vi "DefenderNormalNova.vi"(0 "Enum":T1(ring)=enum."Marcar o mais perigoso", 1 "Atacando contra?":bool=TRUE, 3 "AI Parameters":T9={"GotoKick"={"Dist do cone a frente"=150.0, "attacker farback"=1500.0, "Perto"=300.0, "min dist to kick"=150.0, "kick eps"=0.0, "Time to transition"=0.05}, "Attacker"={"CC chute"=0.09, "CC passe"=0.045, "Kick Force"=100.0, "D ball-robot Kick"=200.0, "D ball-robot Pass"=0.3}, "Defender"={"D max"=1700.0, "Vel p/ robô av"=1000.0, "Kick Force"=100.0, "D atk-def"=0.0, "D farback"=0.0}, "Timeout"={"Field/v in x"=6.0, "Dist Robots"=300, "Dist up in y"=300}, "Pose Striker"={"dist"=200.0, "Numeric"=-4.0, "dist 2"=200.0}, "Dist Stop"=300.0, "Distance when ball out"=200, "D central gap "=150.0, "T pass"=0.0, "Force ++"=0.0, "range kick"=0.0, "Chute alto"=TRUE, "Marcador novo"=TRUE} {"D central gap" format="%#_13g"; "Dist Stop" format="%#_13g"; "Pose Striker"."Numeric" format="%#_13g"; "Defender"."Kick Force" format="%#_13g"; "Defender"."Vel p/ robô av" format="%#_13g"; "Attacker"."D ball-robot Kick" format="%#_13g"; "Attacker"."Kick Force" format="%#_13g"; "Attacker"."CC passe" format="%#_13g"; "Attacker"."CC chute" format="%#_13g"; "GotoKick"."kick eps" format="%#_13g"; "GotoKick"."min dist to kick" format="%#_13g"; "GotoKick"."Perto" format="%#_13g"; "GotoKick"."attacker farback" format="%#_13g"; "GotoKick"."Dist do cone a frente" format="%#_13g"}, 4 "IA State Input 2":T10={"our_robots"=[], "enemy_robots"=[], "balls"=[], "geometry"={"line_width"=0, "field_length"=0, "field_width"=0, "boundary_width"=0, "referee_width"=0, "goal_width"=0, "goal_depth"=0, "goal_wall_width"=0, "center_circle_radius"=0, "defense_radius"=0, "defense_stretch"=0, "free_kick_from_defense_dist"=0, "penalty_spot_from_field_line_dist"=0, "penalty_line_from_spot_dist"=0}, "IA Judge"={"stage"="", "command"="", "our_goalie_id"=0.0, "enemy_goalie_id"=0.0, "command enum"=enum."Halt", "Time"=enum."Azul"}, "Received Timestamp"=timestamp(0 s since 1904-01-01), "Events"={"Touch"=FALSE, "Ball out"=FALSE, "id touch"=0.0, "Ball out of \nVision"=FALSE, "Ball inside \nGoalie area"=FALSE, "Robot not responding"=FALSE, "Robots responding status"=[1.0, 1.0, 1.0, 1.0, 1.0, 1.0], "Enemy Ball \nPossession"=FALSE, "Pass State"=FALSE, "id end of pass"=0.0, "Kick"=FALSE, "Id ini Possession"=0.0, "Ball Possesion"=FALSE, "Id Possesion"=0.0}}, 5 "Stop?":bool, 6 "Defensores":u32[](array[numeric]), 7 "total de \ndefensores":i32, 8 "Field defense":dbl[](array[numeric]), 9 "geometry":T7, 10 "balls":T8[](array[typedef]), 11 "Our Robot":T2={"id"=0, "function"=enum."Attacker", "x"=0.0, "y"=0.0, "orientation"=0.0, "v_tangent"=0.0, "v_normal"=0.0, "v_ang"=0.0, "kick_x"=0.0, "kick_z"=0.0, "dribble"=FALSE, "Timestamp"=timestamp(0 s since 1904-01-01), "estimatives"={"est_v_tangent"=0.0, "est_v_normal"=0.0, "est_vx"=0.0, "est_vy"=0.0, "Pos Robot Est"=[]}, "dest_x_kick"=0.0, "dest_y_kick"=0.0, "Gap Coord"=[], "States"=enum."GoToTangent", "Path "=[], "Path  Smooth"=[], "Dest"=[]}) -> (2 "Robot out":T2={"id"=0, "function"=enum."Attacker", "x"=0.0, "y"=0.0, "orientation"=0.0, "v_tangent"=0.0, "v_normal"=0.0, "v_ang"=0.0, "kick_x"=0.0, "kick_z"=0.0, "dribble"=FALSE, "Timestamp"=timestamp(0 s since 1904-01-01), "estimatives"={"est_v_tangent"=0.0, "est_v_normal"=0.0, "est_vx"=0.0, "est_vy"=0.0, "Pos Robot Est"=[]}, "dest_x_kick"=0.0, "dest_y_kick"=0.0, "Gap Coord"=[], "States"=enum."GoToTangent", "Path "=[], "Path  Smooth"=[], "Dest"=[]})   [LabVIEW 2017]
uses:
  Core/AI Robot.ctl
  Functions Enum.ctl
  AttackerStates.ctl
  Path Planning/RRT/PathDests.ctl
  Path Planning/RRT/PathDest.ctl
  Core/AI Input.ctl
  Core/AI Ball.ctl
  Core/Field Size.ctl
  Core/AI Judge.ctl
  Command Enum.ctl
  Util/Events/Events.ctl
  AI Parameters.ctl
  cb56df22-0c68-485e-ade5-5418ba57ce65.vi
  4d43a6eb-e47f-494e-b5b6-07a2d7f45f03.vi
  <vilib>/Array/Sort 2D Array - Pop Stack.vi
  <vilib>/Array/Sort 2D Array - Push Stack.vi
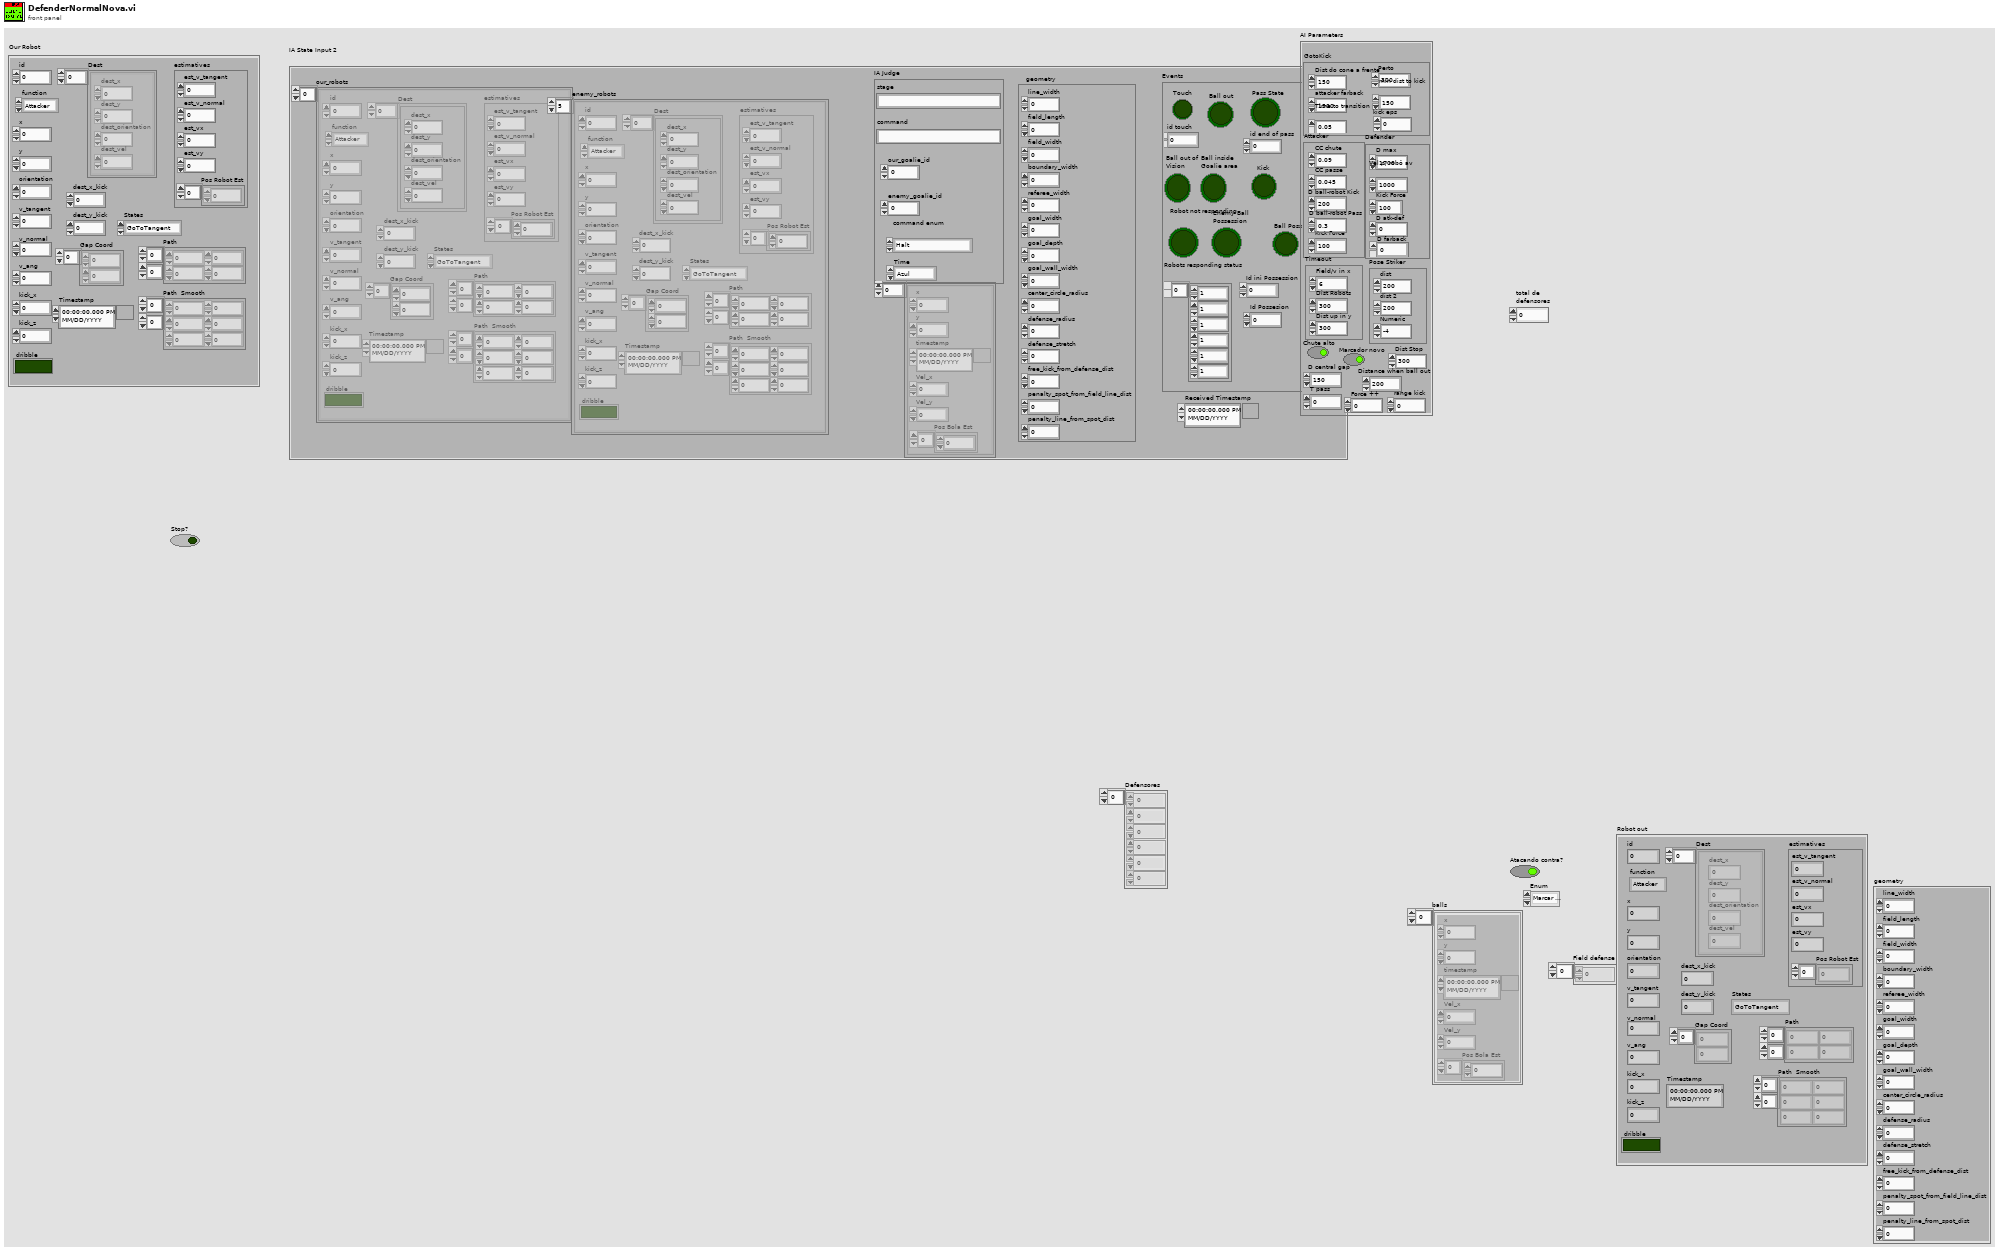
[diagram p1: front panel]
types:
  T1 = enum16{"Marcar Segundo mais perigoso", "Marcar o mais perigoso"}
  T2 = typedef "AI Robot.ctl" = cluster{"id":u32, "function":T3, "x":dbl, "y":dbl, "orientation":dbl, "v_tangent":dbl, "v_normal":dbl, "v_ang":dbl, "kick_x":dbl, "kick_z":dbl, "dribble":bool, "Timestamp":timestamp, "estimatives":cluster{"est_v_tangent":dbl, "est_v_normal":dbl, "est_vx":dbl, "est_vy":dbl, "Pos Robot Est":dbl[]}, "dest_x_kick":dbl, "dest_y_kick":dbl, "Gap Coord":dbl[], "States":T4, "Path ":dbl[][], "Path  Smooth":dbl[][], "Dest":T5}
  T3 = typedef "Functions Enum.ctl" = enum16{"Attacker", "Goalie", "Defender", "Striker", "Goto 0", "Dummy", "Kicker", "ZigZag"}
  T4 = typedef "AttackerStates.ctl" = enum16{"Pass", "GoToTangent", "BallGetting", "GoToKick", ""}
  T5 = typedef "PathDests.ctl" = T6[]
  T6 = typedef "PathDest.ctl" = cluster{"dest_x":dbl, "dest_y":dbl, "dest_orientation":dbl, "dest_vel":dbl}
  T7 = typedef "Field Size.ctl" = cluster{"line_width":u32, "field_length":u32, "field_width":u32, "boundary_width":u32, "referee_width":u32, "goal_width":u32, "goal_depth":u32, "goal_wall_width":u32, "center_circle_radius":u32, "defense_radius":u32, "defense_stretch":u32, "free_kick_from_defense_dist":u32, "penalty_spot_from_field_line_dist":u32, "penalty_line_from_spot_dist":u32}
  T8 = typedef "AI Ball.ctl" = cluster{"x":dbl, "y":dbl, "timestamp":timestamp, "Vel_x":dbl, "Vel_y":dbl, "Pos Bola Est":dbl[]}
  T9 = typedef "AI Parameters.ctl" = cluster{"GotoKick":cluster{"Dist do cone a frente":dbl, "attacker farback":dbl, "Perto":dbl, "min dist to kick":dbl, "kick eps":dbl, "Time to transition":dbl}, "Attacker":cluster{"CC chute":dbl, "CC passe":dbl, "Kick Force":dbl, "D ball-robot Kick":dbl, "D ball-robot Pass":dbl}, "Defender":cluster{"D max":dbl, "Vel p/ robô av":dbl, "Kick Force":dbl, "D atk-def":dbl, "D farback":dbl}, "Timeout":cluster{"Field/v in x":dbl, "Dist Robots":u32, "Dist up in y":u32}, "Pose Striker":cluster{"dist":dbl, "Numeric":dbl, "dist 2":dbl}, "Dist Stop":dbl, "Distance when ball out":i32, "D central gap ":dbl, "T pass":dbl, "Force ++":dbl, "range kick":dbl, "Chute alto":bool, "Marcador novo":bool}
  T10 = typedef "AI Input.ctl" = cluster{"our_robots":T2[], "enemy_robots":T2[], "balls":T8[], "geometry":T7, "IA Judge":T11, "Received Timestamp":timestamp, "Events":T13}
  T11 = typedef "AI Judge.ctl" = cluster{"stage":string, "command":string, "our_goalie_id":dbl, "enemy_goalie_id":dbl, "command enum":T12, "Time":enum16{"Azul", "Amarelo"}}
  T12 = typedef "Command Enum.ctl" = enum16{"Halt", "Stop", "Force Start", "PKA Normal Start", "Prepare Kickoff Ally", "PKE Normal Start", "Prepare Kickoff Enemy", "Prepare Penalty Ally", "PPA Normal Start", "Prepare Penalty Enemy", "PPE Normal Start", "Direct Free Enemy", "Direct Free Ally", "Indirect Free Enemy", "Indirect Free Ally", "Timeout Enemy", "Timeout Ally", "Goal Enemy", "Goal Ally", "Ball Placement Enemy", "Ball Placement Ally", "Normal Half Time", "Extra Time Break", "Extra Half Time", "None", "Post Game"}
  T13 = typedef "Events.ctl" = cluster{"Touch":bool, "Ball out":bool, "id touch":dbl, "Ball out of \nVision":bool, "Ball inside \nGoalie area":bool, "Robot not responding":bool, "Robots responding status":dbl[], "Enemy Ball \nPossession":bool, "Pass State":bool, "id end of pass":dbl, "Kick":bool, "Id ini Possession":dbl, "Ball Possesion":bool, "Id Possesion":dbl}
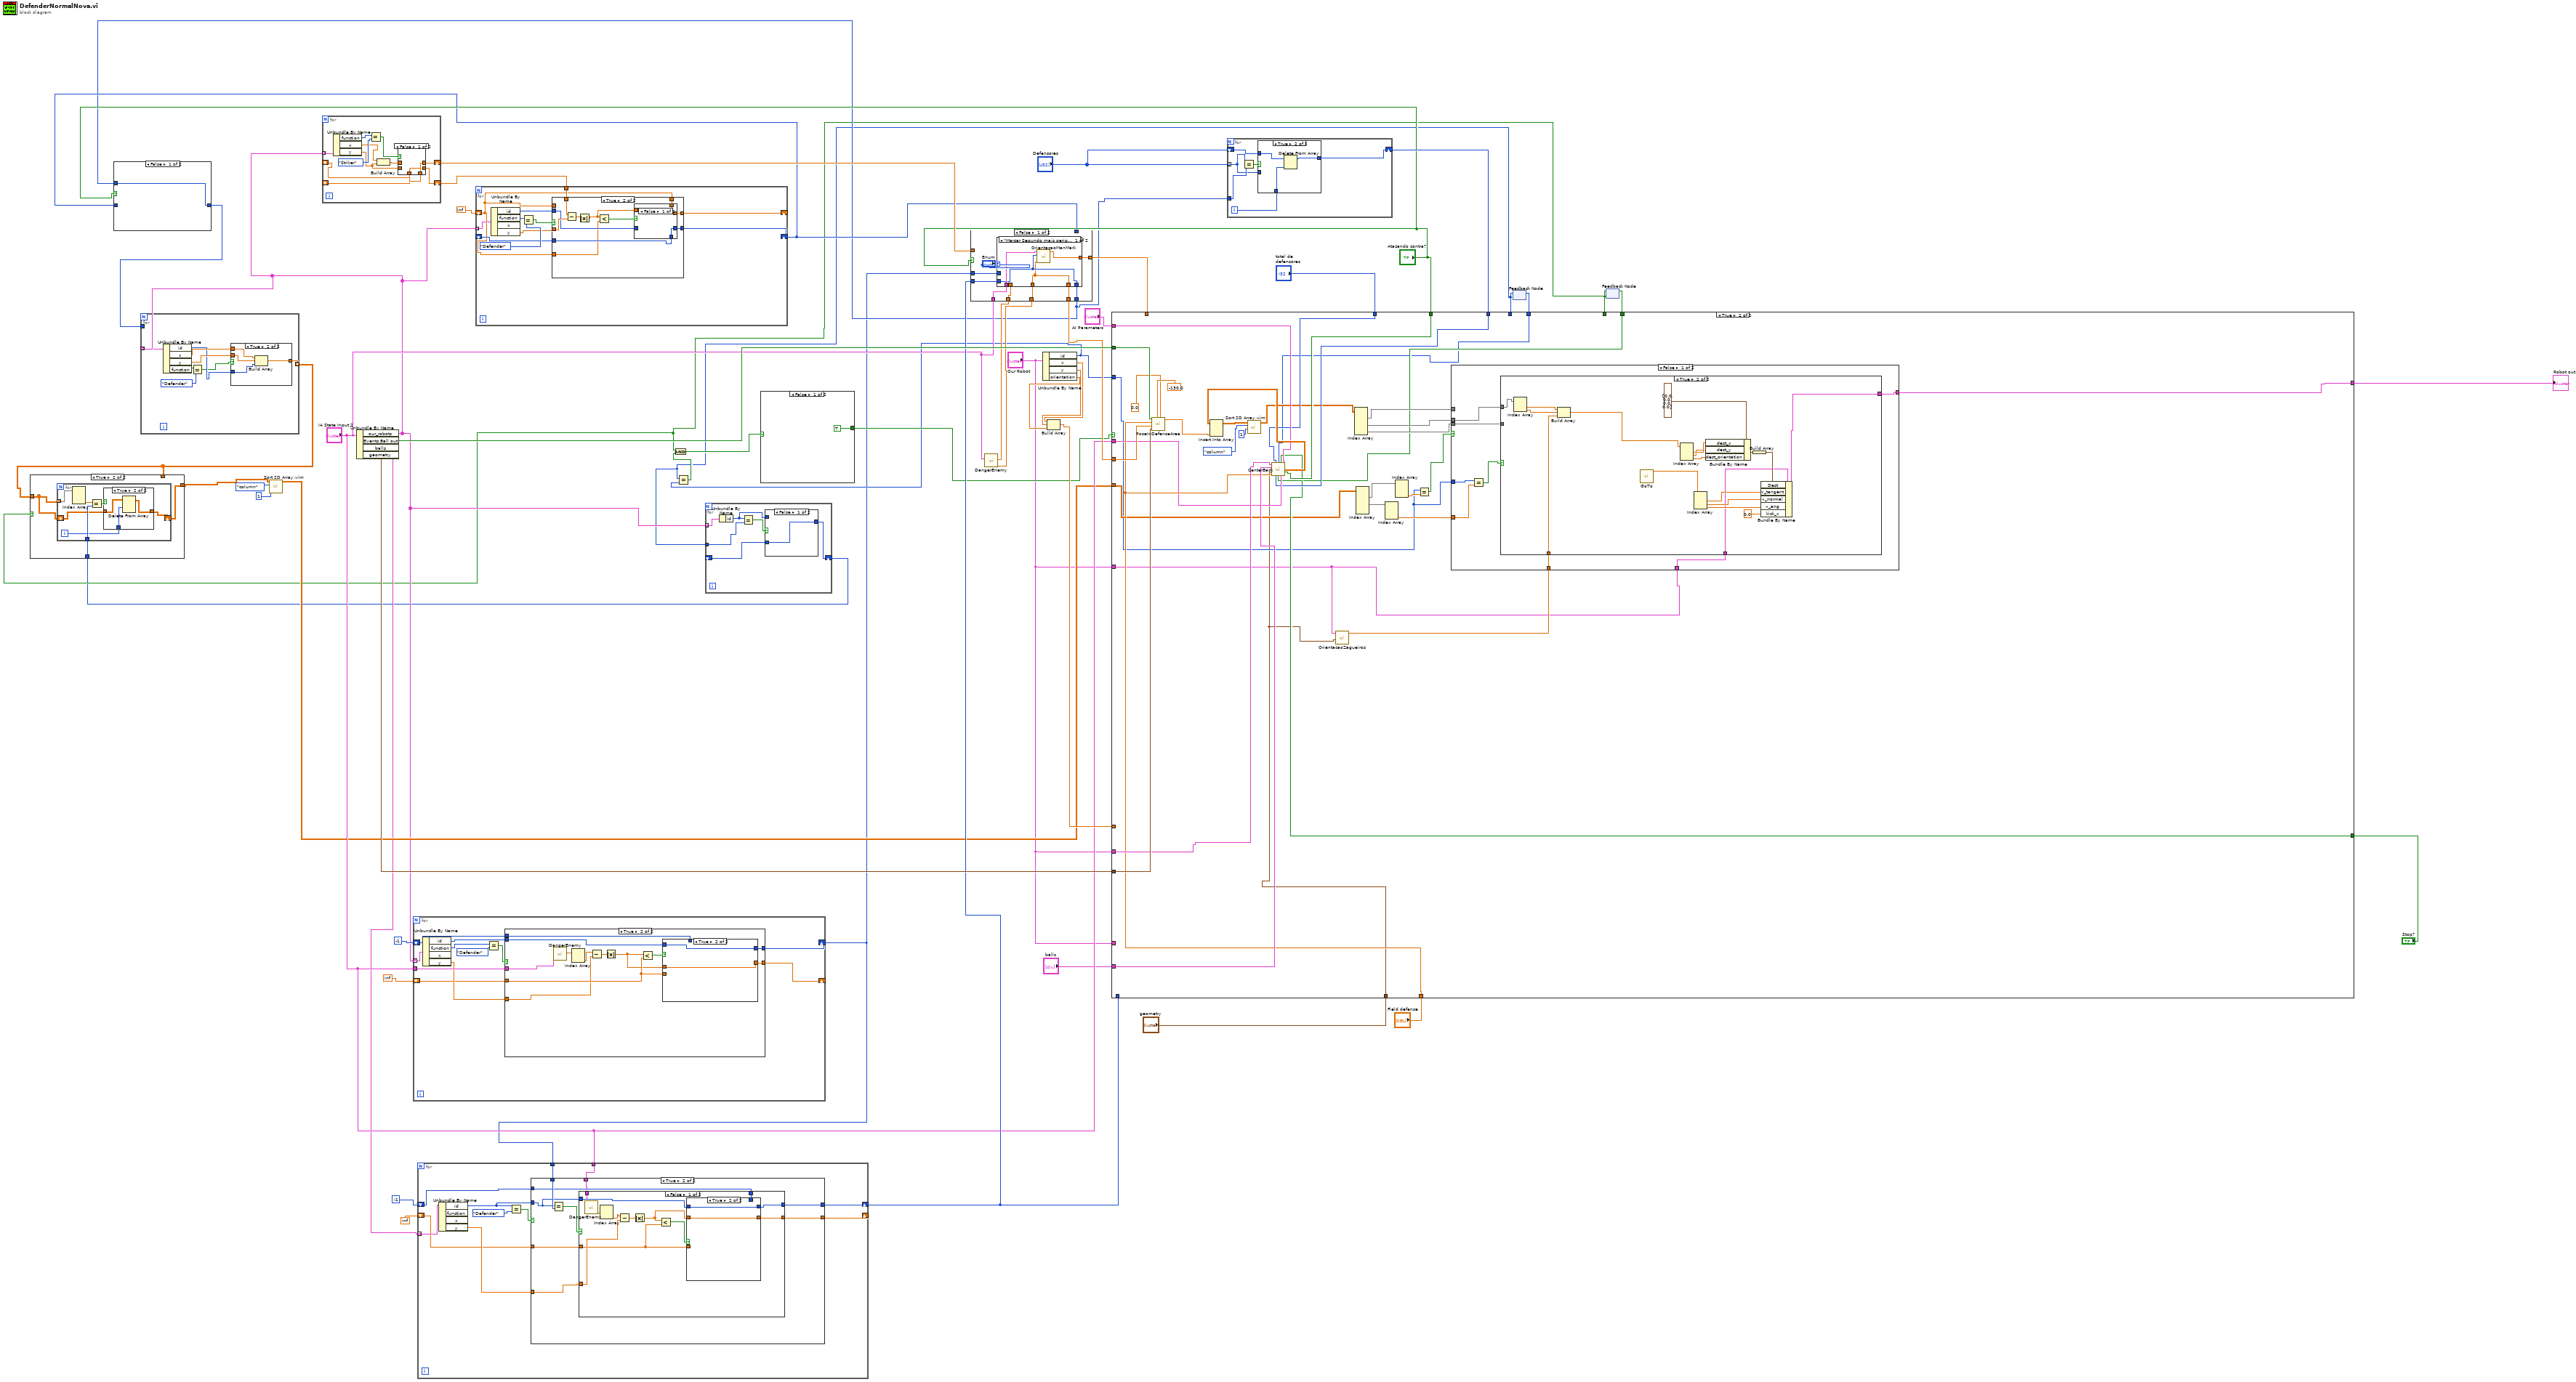
[diagram p0: block diagram]
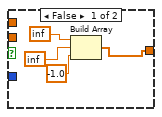
[diagram p6: hidden frame]
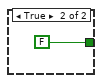
[diagram p7: hidden frame]
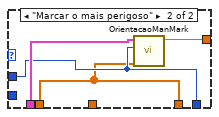
[diagram p11: hidden frame]
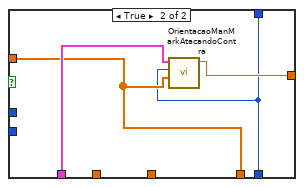
[diagram p12: hidden frame]
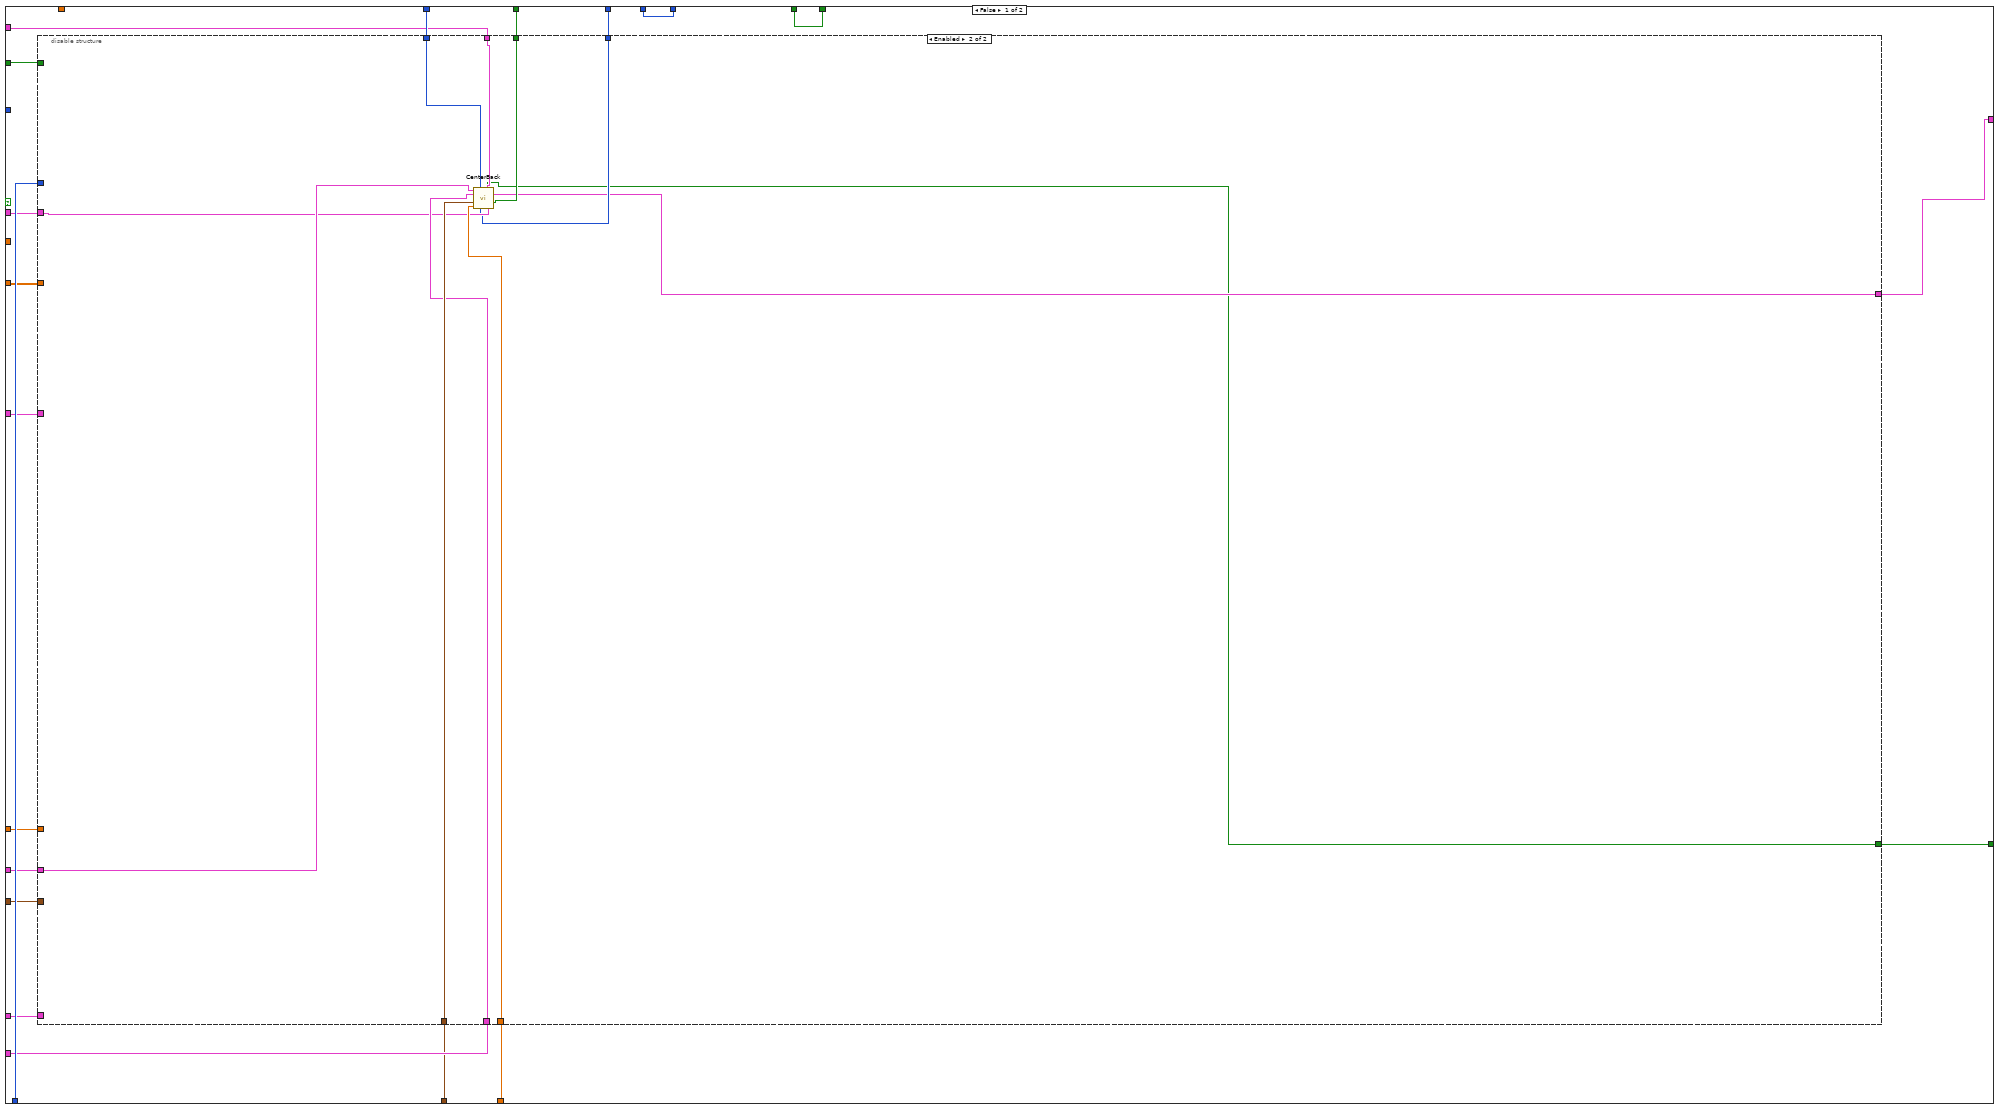
[diagram p17: hidden frame]
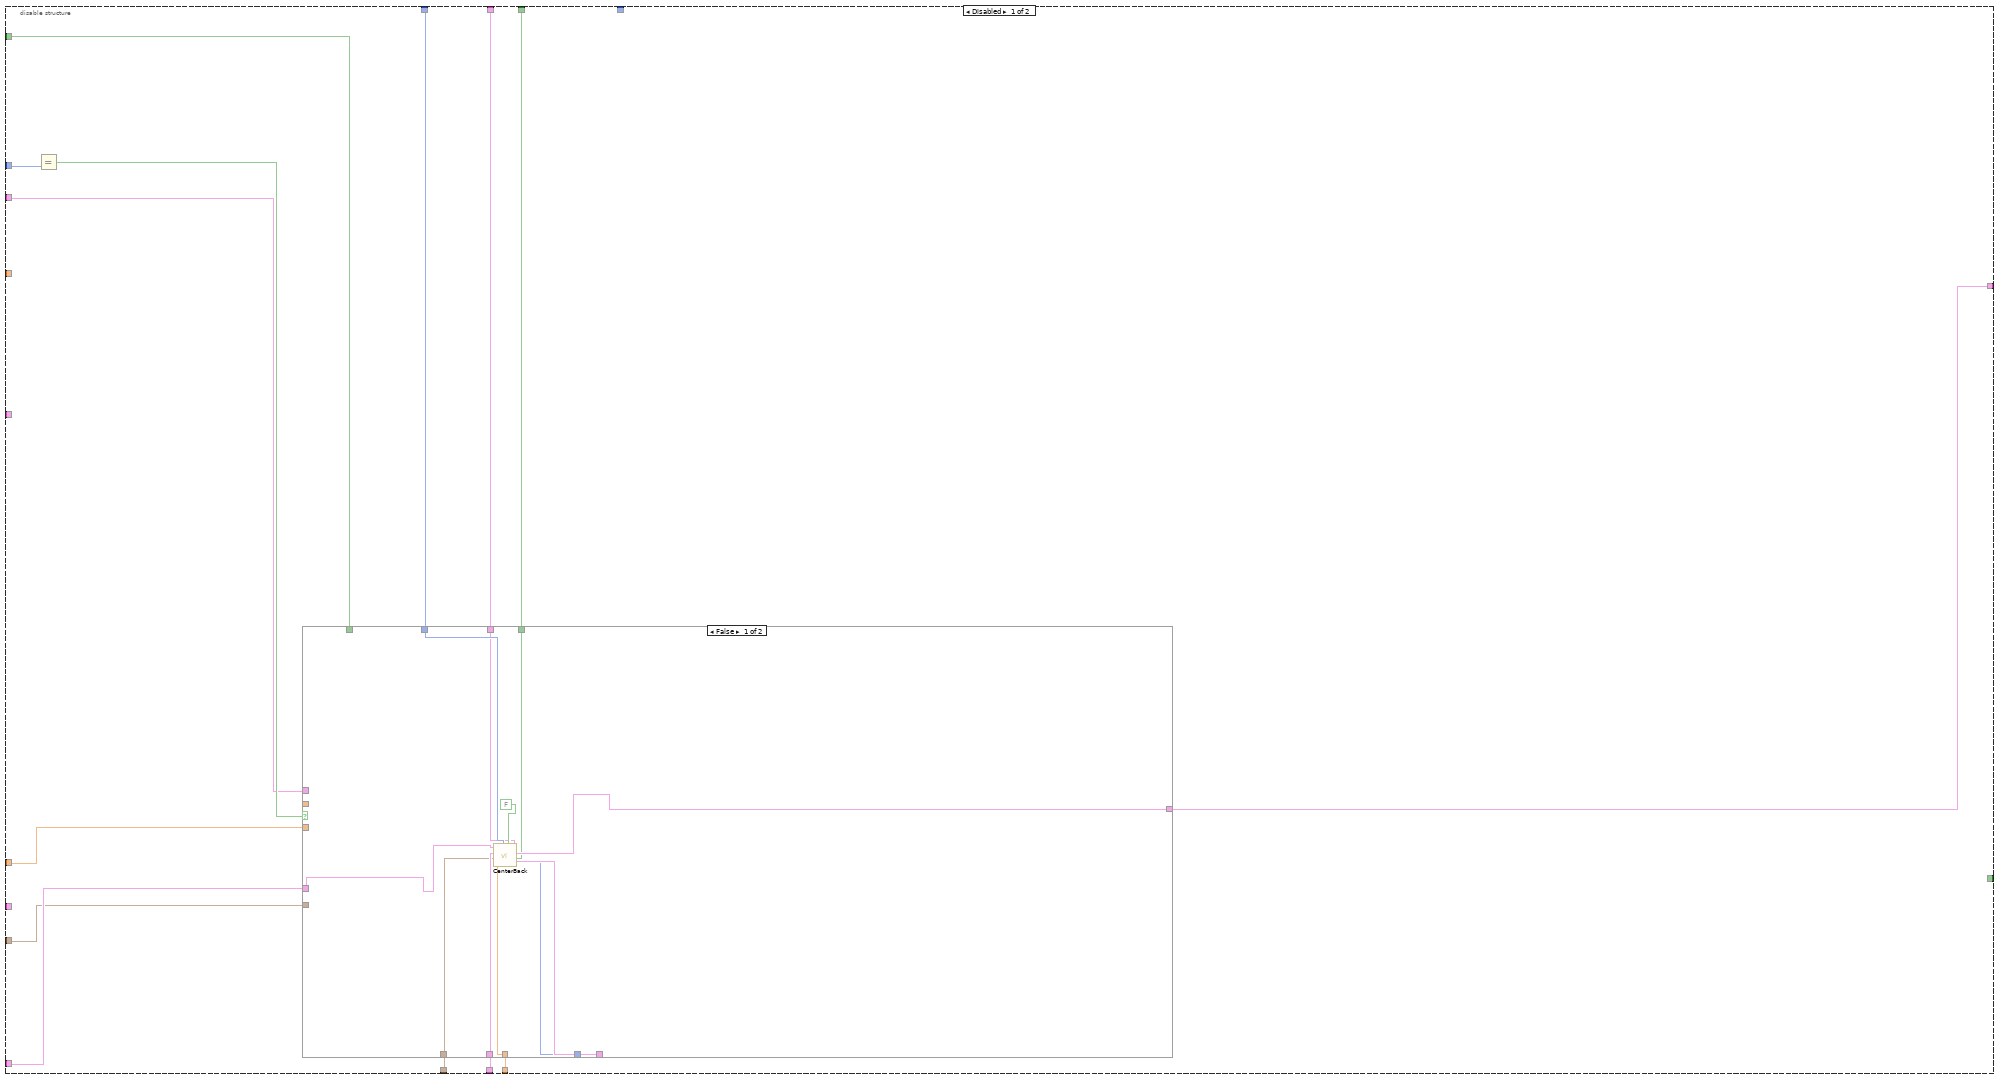
[diagram p18: hidden frame]
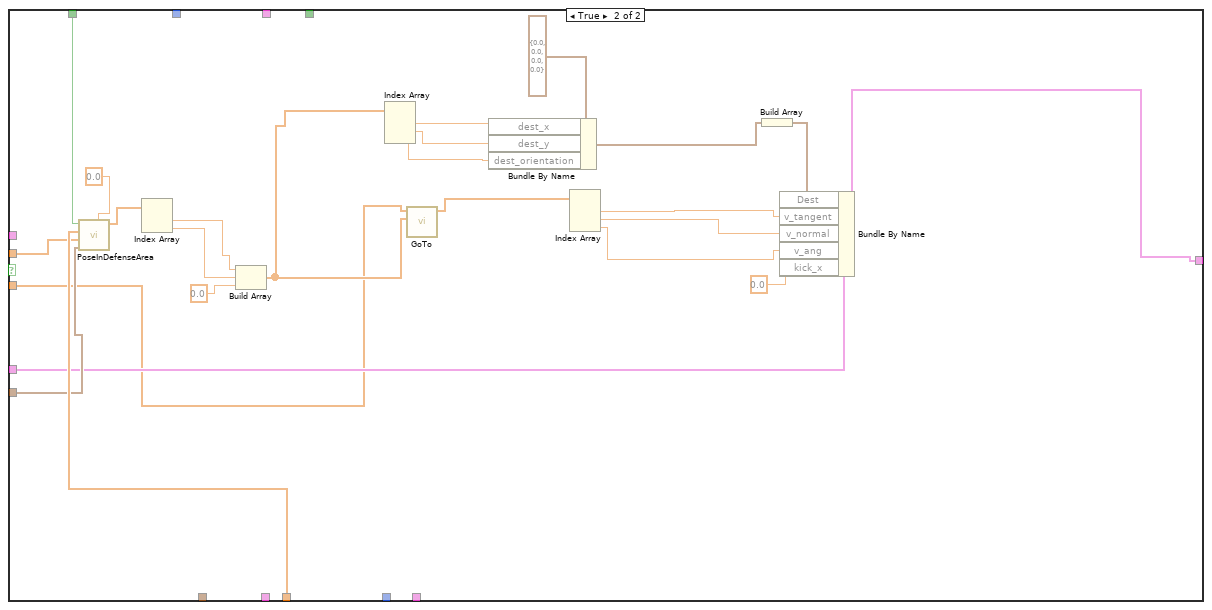
[diagram p19: hidden frame]
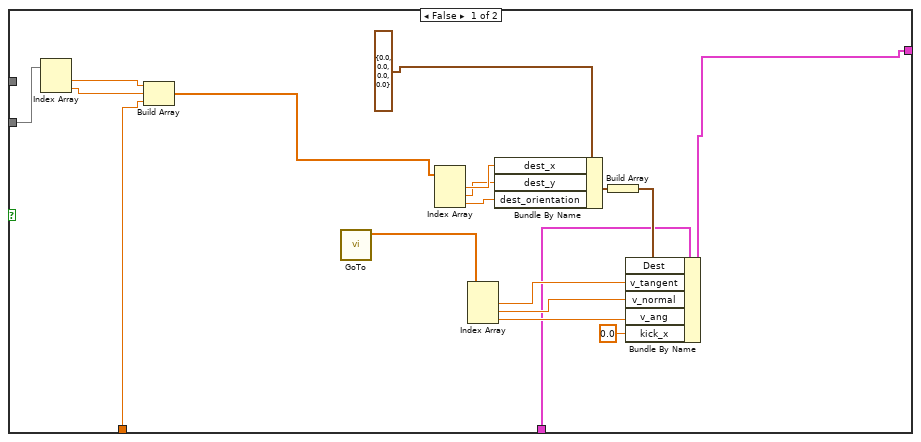
[diagram p20: hidden frame]
diagram:
  n1 = Unbundle By Name("IA State Input 2") -> ("our_robots"=w7:T2[], "Events.Ball out"=w44:bool, "geometry"=w45:T7)  [unwired: 1 out]
  n2 = for {
    tunnel: w7 -> [w60] mode=indexing
    shift-right: [w54] -> w32
    shift-left: _ -> [w53]
    shift-right: [w51] -> w20
    shift-left: _ -> [w50]
    n3 = Unbundle By Name(w60) -> ("function"=w59:T3, "x"=w56:dbl, "y"=w52:dbl)
    n4 = Equal?(x=w59, y=Functions_Enum."Striker" ("x")) -> (x = y?=w57:bool)
    n5 = Build Array(w56, w52) -> (w55:dbl[])
    n6 = case shown="False" w57 {
      tunnel: w55 -> [_ w64]
      tunnel: [w62 w64] -> w54
      tunnel: w53 -> [w62 _]
      tunnel: [w61 w63] -> w51
      tunnel: w52 -> [_ w63]
      tunnel: w50 -> [w61 _]
      frame False {
      }
      frame True {
      }
    }
  }
  n7 = for {
    tunnel: w7 -> [w75] mode=indexing
    tunnel: "IA State Input 2" -> [w71]
    shift-right: [w68] -> w1
    shift-left: -1 -> [w65]
    shift-right: [w67] -> _
    shift-left: inf -> [w66]
    n8 = Unbundle By Name(w75) -> ("id"=w69:u32, "function"=w74:T3, "y"=w70:dbl)  [unwired: 1 out]
    n9 = Equal?(x=w74, y=Functions_Enum."Defender" ("x")) -> (x = y?=w72:bool)
    n10 = case shown="True" w72 {
      tunnel: w71 -> [_ w89]
      tunnel: w70 -> [_ w80]
      tunnel: w69 -> [_ w87]
      tunnel: [w77 w86] -> w68
      tunnel: [w76 w85] -> w67
      tunnel: w66 -> [w76 w84]
      tunnel: w65 -> [w77 w83]
      frame False {
      }
      frame True {
        n11 = call "DangerEnemy.vi"("IA Input"=w89) -> ("Pos do inimigo\nperigoso"=w82:dbl[])  [unwired: 7 in, 3 out]
        n12 = Index Array(array=w82) -> (element #2=w81:dbl)  [unwired: 2 in, 1 out]
        n13 = Subtract(x=w81, y=w80) -> (x-y=w79:dbl)
        n14 = Absolute Value(x=w79) -> (abs(x)=w78:dbl)
        n15 = Less?(x=w78, y=w84) -> (x < y?=w88:bool)
        n16 = case shown="True" w88 {
          tunnel: w87 -> [_ w93]
          tunnel: [w90 w93] -> w86
          tunnel: [w91 w92] -> w85
          tunnel: w78 -> [_ w92]
          tunnel: w84 -> [w91 _]
          tunnel: w83 -> [w90 _]
          frame False {
          }
          frame True {
          }
        }
      }
    }
  }
  n17 = for {
    tunnel: w7 -> [w104] mode=indexing
    tunnel: w1 -> [w100]
    shift-right: [w98] -> _
    shift-left: inf -> [w95]
    shift-right: [w97] -> w33
    shift-left: -1 -> [w96]
    tunnel: "IA State Input 2" -> [w94]
    n18 = Unbundle By Name(w104) -> ("id"=w101:u32, "y"=w99:dbl)  [unwired: 2 out]
    n19 = Equal?(x=w101, y=Functions_Enum."Defender" ("x")) -> (x = y?=w102:bool)
    n20 = case shown="True" w102 {
      tunnel: w101 -> [_ w111]
      tunnel: w100 -> [_ w115]
      tunnel: w99 -> [_ w108]
      tunnel: [w105 w113] -> w98
      tunnel: [w106 w112] -> w97
      tunnel: w96 -> [w106 w110]
      tunnel: w95 -> [w105 w109]
      tunnel: w94 -> [_ w107]
      frame False {
      }
      frame True {
        n21 = Equal?(x=w111, y=w115) -> (x = y?=w114:bool)
        n22 = case shown="False" w114 {
          tunnel: w108 -> [w118 _]
          tunnel: [w126 w132] -> w113
          tunnel: [w124 w133] -> w112
          tunnel: w111 -> [w125 _]
          tunnel: w110 -> [w123 w133]
          tunnel: w109 -> [w122 w132]
          tunnel: w107 -> [w121 _]
          frame False {
            n23 = call "DangerEnemy.vi"("IA Input"=w121) -> ("Pos do segundo inimigo\nperigoso"=w120:dbl[])  [unwired: 7 in, 3 out]
            n24 = Index Array(array=w120) -> (element #2=w119:dbl)  [unwired: 2 in, 1 out]
            n25 = Subtract(x=w119, y=w118) -> (x-y=w117:dbl)
            n26 = Absolute Value(x=w117) -> (abs(x)=w116:dbl)
            n27 = Less?(x=w116, y=w122) -> (x < y?=w127:bool)
            n28 = case shown="True" w127 {
              tunnel: [w128 w131] -> w126
              tunnel: w116 -> [_ w131]
              tunnel: [w129 w130] -> w124
              tunnel: w125 -> [_ w130]
              tunnel: w123 -> [w129 _]
              tunnel: w122 -> [w128 _]
              frame False {
              }
              frame True {
              }
            }
          }
          frame True {
          }
        }
      }
    }
  }
  n29 = for {
    tunnel: w7 -> [w144] mode=indexing
    tunnel: w20 -> [w140]
    shift-right: [w139] -> _
    shift-left: inf -> [w135]
    shift-right: [w137] -> w14
    shift-left: _ -> [w136]
    n30 = Unbundle By Name(w144) -> ("id"=w138:u32, "function"=w143:T3, "y"=w134:dbl)  [unwired: 1 out]
    n31 = Equal?(x=w143, y=Functions_Enum."Defender") -> (x = y?=w141:bool)
    n32 = case shown="True" w141 {
      tunnel: w134 -> [_ w157]
      tunnel: w140 -> [_ w156]
      tunnel: [w146 w154] -> w139
      tunnel: w138 -> [_ w153]
      tunnel: [w145 w152] -> w137
      tunnel: w136 -> [w145 w151]
      tunnel: w135 -> [_ w150]
      tunnel: w135 -> [w146 _]
      tunnel: w135 -> [_ w149]
      frame False {
      }
      frame True {
        n33 = Subtract(x=w156, y=w157) -> (x-y=w148:dbl)
        n34 = Absolute Value(x=w148) -> (abs(x)=w147:dbl)
        n35 = Less?(x=w147, y=w149) -> (x < y?=w155:bool)
        n36 = case shown="False" w155 {
          tunnel: w147 -> [_ w161]
          tunnel: [w158 w161] -> w154
          tunnel: w153 -> [_ w160]
          tunnel: [w159 w160] -> w152
          tunnel: w151 -> [w159 _]
          tunnel: w150 -> [w158 _]
          frame False {
          }
          frame True {
          }
        }
      }
    }
  }
  n37 = call "DangerEnemy.vi"("IA Input"="IA State Input 2") -> ("Pos do segundo inimigo\nperigoso"=w35:dbl[], "Pos do inimigo\nperigoso"=w36:dbl[])  [unwired: 7 in, 2 out]
  n38 = case shown="False" "Atacando contra?" {
    tunnel: w32 -> [_ w181]
    tunnel: [w168 w181] -> w37
    tunnel: w36 -> [w169 _]
    tunnel: w35 -> [w167 _]
    tunnel: w1 -> [w166 _]
    tunnel: [w165 w179] -> w13
    tunnel: w33 -> [w164 _]
    tunnel: w14 -> [_ w179]
    tunnel: "IA State Input 2" -> [w163 w182]
    tunnel: [w162 w180] -> w27
    frame False {
      n39 = case shown="\"Marcar Segundo mais perigoso\", Default" "Enum" {
        tunnel: w169 -> [_ w175]
        tunnel: [w171 w175] -> w168
        tunnel: w167 -> [w171 _]
        tunnel: [w173 w177] -> w165
        tunnel: w166 -> [_ w177]
        tunnel: w164 -> [w173 _]
        tunnel: w163 -> [w174 w178]
        tunnel: [w172 w176] -> w162
        frame "Marcar Segundo mais perigoso", Default {
          n40 = call "OrientacaoManMark.vi"("Pos inimigo perigoso"=w171, "Id ManMark"=w173, "IA State Input 2"=w174) -> ("Orientacao ManMark"=w172:dbl)  [unwired: 8 in]
        }
        frame "Marcar o mais perigoso" {
          n41 = call "OrientacaoManMark.vi"("Pos inimigo perigoso"=w175, "Id ManMark"=w177, "IA State Input 2"=w178) -> ("Orientacao ManMark"=w176:dbl)  [unwired: 8 in]
        }
      }
    }
    frame True {
      n42 = call "OrientacaoManMarkAtacandoContra.vi"("Pos striker"=w181, "Id ManMark"=w179, "IA State Input 2"=w182) -> ("Orientacao ManMark"=w180:dbl)  [unwired: 8 in]
    }
  }
  n43 = case shown="False" "Atacando contra?" {
    tunnel: w14 -> [_ w184]
    tunnel: [w183 w184] -> w12
    tunnel: w13 -> [w183 _]
    frame False {
    }
    frame True {
    }
  }
  n44 = for {
    tunnel: w7 -> [w192] mode=indexing
    tunnel: [w187] -> w3 mode=indexing
    tunnel: w12 -> [_]
    n45 = Unbundle By Name(w192) -> ("id"=w186:u32, "x"=w189:dbl, "y"=w188:dbl, "function"=w191:T3)
    n46 = Equal?(x=w191, y=Functions_Enum."Defender") -> (x = y?=w185:bool)
    n47 = case shown="True" w185 {
      tunnel: w189 -> [_ w200]
      tunnel: w188 -> [_ w199]
      tunnel: w186 -> [_ w198]
      tunnel: [w193 w197] -> w187
      frame False {
        n48 = Build Array(inf ("element"), inf ("element"), -1.0 ("element")) -> (w193:dbl[])
      }
      frame True {
        n49 = Build Array(w200, w199, w198) -> (w197:dbl[])
      }
    }
  }
  n50 = Unbundle By Name("Our Robot") -> ("id"=w8:u32, "x"=w43:dbl, "y"=w42:dbl, "orientation"=w41:dbl)
  n51 = Build Array(w43, w42, w41) -> (w40:dbl[])
  n52 = for {
    tunnel: "Defensores" -> [w201] mode=indexing
    tunnel: w13 -> [w204]
    shift-right: [w203] -> w30
    shift-left: "Defensores" -> [w202]
    i -> [w205]
    n53 = Equal?(x=w201, y=w204) -> (x = y?=w206:bool)
    n54 = case shown="True" w206 {
      tunnel: w202 -> [w207 w209]
      tunnel: w205 -> [_ w208]
      tunnel: [w207 w210] -> w203
      tunnel: w201 -> [_ _]
      frame False {
      }
      frame True {
        n55 = Delete From Array(array=w209, index=w208) -> (array with subset deleted=w210:u32[])  [unwired: 1 in, 1 out]
      }
    }
  }
  n56 = feedback #1() -> (w6:i32)  [unwired: 1 in]
  n57 = Equal?(x=w6, y=w8) -> (x = y?=w24:bool)
  n58 = for {
    tunnel: w7 -> [w216] mode=indexing
    tunnel: w6 -> [w215]
    shift-right: [w212] -> w2
    shift-left: _ -> [w211]
    n59 = Unbundle By Name(w216) -> ("id"=w213:u32)
    n60 = Equal?(x=w213, y=w215) -> (x = y?=w214:bool)
    n61 = case shown="False" w214 {
      tunnel: w213 -> [_ w218]
      tunnel: [w217 w218] -> w212
      tunnel: w211 -> [w217 _]
      frame False {
      }
      frame True {
      }
    }
  }
  n62 = feedback #2() -> (w5:bool)  [unwired: 1 in]
  n63 = case shown="True" w5 {
    tunnel: [w219 w220] -> w4
    tunnel: w3 -> [w219 _]
    tunnel: w3 -> [_ w221]
    tunnel: w2 -> [_ w222]
    frame False {
    }
    frame True {
      n64 = for {
        tunnel: w221 -> [w229] mode=indexing
        tunnel: w222 -> [w227]
        shift-right: [w224] -> w220
        shift-left: w221 -> [w223]
        i -> [w225]
        n65 = Index Array(array=w229) -> (element #3=w228:dbl)  [unwired: 3 in, 2 out]
        n66 = Equal?(x=w228, y=w227) -> (x = y?=w226:bool)
        n67 = case shown="True" w226 {
          tunnel: w223 -> [w230 w233]
          tunnel: w225 -> [_ w232]
          tunnel: [w230 w231] -> w224
          frame False {
          }
          frame True {
            n68 = Delete From Array(array=w233, index (row)=w232) -> (array with subset deleted=w231:dbl[][])  [unwired: 2 in, 1 out]
          }
        }
      }
    }
  }
  n69 = call "Sort 2D Array.vim"("index"=1, "dimension to index (column)"=enum16{"column", "row"}."column", "2D array"=w4) -> ("sorted 2D array"=w17:dbl[][])  [unwired: 7 in, 1 out]
  n70 = And(x=w5, y=w24) -> (x .and. y?=w23:bool)
  n71 = case shown="False" w23 {
    tunnel: [TRUE FALSE] -> w22
    frame False {
    }
    frame True {
    }
  }
  n72 = case shown="True" w22 {
    tunnel: "IA State Input 2" -> [w253 w338]
    tunnel: "Our Robot" -> [w254 _]
    tunnel: w8 -> [_ w326]
    tunnel: w33 -> [w255 _]
    tunnel: [w242 w329] -> w21
    tunnel: w45 -> [w251 w353]
    tunnel: w44 -> [w252 w352]
    tunnel: w40 -> [w250 _]
    tunnel: "Our Robot" -> [w244 w344]
    tunnel: w37 -> [_ w351]
    tunnel: "total de \ndefensores" -> [w249 w336]
    tunnel: "Atacando contra?" -> [w248 w339]
    tunnel: "AI Parameters" -> [w247 w340]
    tunnel: "balls" -> [w246 w343]
    tunnel: "geometry" -> [w245 w322]
    tunnel: "Field defense" -> [w243 w342]
    tunnel: "Stop?" -> [w241 w335]
    tunnel: w30 -> [w240 w337]
    tunnel: w27 -> [_ _]
    tunnel: [w237 w318] -> w26
    tunnel: w6 -> [w237 _]
    tunnel: [w236 w319] -> w25
    tunnel: w5 -> [w236 _]
    tunnel: w17 -> [w239 w333]
    tunnel: "Our Robot" -> [w238 w320]
    frame False {
      n73 = disable-structure shown="Enabled" {
        disable-tunnel: w255 -> [w270 _]
        disable-tunnel: w254 -> [w268 _]
        disable-tunnel: w253 -> [w267 w313]
        disable-tunnel: [w266 w308] -> w242
        disable-tunnel: w243 -> [w265 w315]
        disable-tunnel: w252 -> [w264 _]
        disable-tunnel: w251 -> [w263 _]
        disable-tunnel: w250 -> [w261 _]
        disable-tunnel: w249 -> [w260 w310]
        disable-tunnel: w248 -> [w259 w311]
        disable-tunnel: w247 -> [w258 w309]
        disable-tunnel: w246 -> [w257 w314]
        disable-tunnel: w245 -> [w256 w316]
        disable-tunnel: w244 -> [_ w317]
        disable-tunnel: w241 -> [_ w307]
        disable-tunnel: w240 -> [_ w312]
        disable-tunnel: w239 -> [_ _]
        disable-tunnel: w238 -> [_ _]
        frame Disabled {
          n74 = Equal?(y=w270) -> (x=w271:u32, x = y?=w269:bool)
          n75 = case shown="False" w269 {
            tunnel: _ -> [w281 _]
            tunnel: w268 -> [w280 w286]
            tunnel: w267 -> [_ _]
            tunnel: [w279 w284] -> w266
            tunnel: w265 -> [w278 w305]
            tunnel: w264 -> [_ w306]
            tunnel: w263 -> [_ w304]
            tunnel: [_ w303] -> w262
            tunnel: w261 -> [_ w285]
            tunnel: w260 -> [w277 _]
            tunnel: w259 -> [w276 _]
            tunnel: w258 -> [w275 _]
            tunnel: w257 -> [w274 _]
            tunnel: w256 -> [w273 _]
            tunnel: _ -> [w272 _]
            frame False {
              n76 = call "CenterBack.vi"("Atacando contra?"=w276, "AI Parameters"=w275, "IA State Input 2"=w281, "Stop?"=FALSE, "Defensores"=w272, "total"=w277, "Field defense"=w278, "Field Size in"=w273, "balls"=w274, "Our Robot in"=w280) -> ("Robot out"=w279:T2)  [unwired: 1 in]
            }
            frame True {
              n77 = call "PoseInDefenseArea.vi"("theta"=0.0, "geometry"=w304, "Ball"=w303, "Field defense"=w305, "Events.Ball out"=w306) -> ("Array"=w289:dbl[])  [unwired: 6 in]
              n78 = Index Array(array=w289) -> (element #1=w288:dbl, element #2=w287:dbl)  [unwired: 2 in]
              n79 = Build Array(w288, w287, 0.0 ("element")) -> (w300:dbl[])
              n80 = Index Array(array=w300) -> (element #1=w298:dbl, element #2=w297:dbl, element #3=w296:dbl)  [unwired: 3 in]
              n81 = call "GoTo.vi"("Target"=w300, "Position"=w285) -> ("Output\nVelocity"=w301:dbl[])  [unwired: 8 in, 1 out]
              n82 = Bundle By Name(cluster=T6 {"dest_x"=0.0, "dest_y"=0.0, "dest_orientation"=0.0, "dest_vel"=0.0} ("element"), "dest_x"=w298, "dest_y"=w297, "dest_orientation"=w296) -> (w294:T6)
              n83 = Index Array(array=w301) -> (element #1=w293:dbl, element #2=w292:dbl, element #3=w291:dbl)  [unwired: 3 in]
              n84 = Build Array(w294) -> (w295:T6[])
              n85 = Bundle By Name(cluster=w286, "Dest"=w295, "v_tangent"=w293, "v_normal"=w292, "v_ang"=w291, "kick_x"=0.0) -> (w284:T2)
            }
          }
        }
        frame Enabled {
          n86 = call "CenterBack.vi"("Our Robot in"=w317, "total"=w310, "Stop?"=w307, "AI Parameters"=w309, "balls"=w314, "Field Size in"=w316, "Atacando contra?"=w311, "Field defense"=w315, "Defensores"=w312, "IA State Input 2"=w313) -> ("Robot out"=w308:T2)  [unwired: 2 in, 3 out]
        }
      }
    }
    frame True {
      n87 = call "PoseInDefenseArea.vi"("theta"=0.0, "Recuo"=-130.0, "geometry"=w353, "Ball"=w351, "Field defense"=w342, "Events.Ball out"=w352) -> ("Array"=w348:dbl[])  [unwired: 5 in]
      n88 = call "CenterBack.vi"("Our Robot in"=w344, "total"=w336, "Stop?"=w335, "AI Parameters"=w340, "balls"=w343, "Field Size in"=w322, "Atacando contra?"=w339, "Field defense"=w342, "Defensores"=w337, "IA State Input 2"=w338) -> ("Id duelist"=w318:i32, "Pos Centers Back"=w341:dbl[][], "Zageuiro duelist?"=w319:bool)  [unwired: 2 in, 1 out]
      n89 = Insert Into Array(array=w341, new element=w348) -> (w347:dbl[][])  [unwired: 2 in]
      n90 = call "Sort 2D Array.vim"("index"=1, "dimension to index (column)"=enum16{"column", "row"}."column", "2D array"=w347) -> ("sorted 2D array"=w334:dbl[][])  [unwired: 7 in, 1 out]
      n91 = call "OrientacaoZagueiros.vi"("geometry"=w322, "Our Robot"=w320) -> ("Orientação Center Back"=w321:dbl)  [unwired: 9 in]
      n92 = Index Array(array=w334) -> (element #1=w325:dbl[], element #2=w324:dbl[], element #3=w323:dbl[])  [unwired: 6 in]
      n93 = Index Array(array=w333) -> (element #1=w332:dbl[], element #2=w328:dbl[])  [unwired: 6 in, 1 out]
      n94 = Index Array(array=w328) -> (element #3=w327:dbl)  [unwired: 3 in, 2 out]
      n95 = Index Array(array=w332) -> (element #3=w331:dbl)  [unwired: 3 in, 2 out]
      n96 = Equal?(x=w326, y=w331) -> (x = y?=w330:bool)
      n97 = case shown="False" w330 {
        tunnel: w320 -> [w358 w405]
        tunnel: [w357 w404] -> w329
        tunnel: w327 -> [w361 _]
        tunnel: w326 -> [w360 _]
        tunnel: w325 -> [_ w402]
        tunnel: w324 -> [w356 _]
        tunnel: w323 -> [w355 _]
        tunnel: w321 -> [w354 w398]
        frame False {
          n98 = Equal?(x=w360, y=w361) -> (x = y?=w359:bool)
          n99 = case shown="True" w359 {
            tunnel: w358 -> [w366 w386]
            tunnel: [w367 w385] -> w357
            tunnel: w356 -> [_ w382]
            tunnel: w355 -> [w365 _]
            tunnel: w354 -> [w362 w380]
            frame False {
              n100 = Index Array(array=w365) -> (element #1=w369:dbl, element #2=w368:dbl)  [unwired: 2 in]
              n101 = Build Array(w369, w368, w362) -> (w370:dbl[])
              n102 = call "GoTo.vi"() -> ("Output\nVelocity"=w379:dbl[])  [unwired: 10 in, 1 out]
              n103 = Index Array(array=w370) -> (element #1=w375:dbl, element #2=w374:dbl, element #3=w373:dbl)  [unwired: 3 in]
              n104 = Index Array(array=w379) -> (element #1=w376:dbl, element #2=w378:dbl, element #3=w377:dbl)  [unwired: 3 in]
              n105 = Bundle By Name(cluster=T6 {"dest_x"=0.0, "dest_y"=0.0, "dest_orientation"=0.0, "dest_vel"=0.0} ("element"), "dest_x"=w375, "dest_y"=w374, "dest_orientation"=w373) -> (w372:T6)
              n106 = Build Array(w372) -> (w371:T6[])
              n107 = Bundle By Name(cluster=w366, "Dest"=w371, "v_tangent"=w376, "v_normal"=w378, "v_ang"=w377, "kick_x"=0.0) -> (w367:T2)
            }
            frame True {
              n108 = Index Array(array=w382) -> (element #1=w384:dbl, element #2=w383:dbl)  [unwired: 2 in]
              n109 = Build Array(w384, w383, w380) -> (w387:dbl[])
              n110 = call "GoTo.vi"() -> ("Output\nVelocity"=w397:dbl[])  [unwired: 10 in, 1 out]
              n111 = Index Array(array=w387) -> (element #1=w392:dbl, element #2=w391:dbl, element #3=w390:dbl)  [unwired: 3 in]
              n112 = Index Array(array=w397) -> (element #1=w394:dbl, element #2=w396:dbl, element #3=w395:dbl)  [unwired: 3 in]
              n113 = Bundle By Name(cluster=T6 {"dest_x"=0.0, "dest_y"=0.0, "dest_orientation"=0.0, "dest_vel"=0.0} ("element"), "dest_x"=w392, "dest_y"=w391, "dest_orientation"=w390) -> (w389:T6)
              n114 = Build Array(w389) -> (w388:T6[])
              n115 = Bundle By Name(cluster=w386, "Dest"=w388, "v_tangent"=w394, "v_normal"=w396, "v_ang"=w395, "kick_x"=0.0) -> (w385:T2)
            }
          }
        }
        frame True {
          n116 = Index Array(array=w402) -> (element #1=w401:dbl, element #2=w400:dbl)  [unwired: 2 in]
          n117 = Build Array(w401, w400, w398) -> (w403:dbl[])
          n118 = call "GoTo.vi"() -> ("Output\nVelocity"=w415:dbl[])  [unwired: 10 in, 1 out]
          n119 = Index Array(array=w403) -> (element #1=w410:dbl, element #2=w409:dbl, element #3=w408:dbl)  [unwired: 3 in]
          n120 = Index Array(array=w415) -> (element #1=w412:dbl, element #2=w414:dbl, element #3=w413:dbl)  [unwired: 3 in]
          n121 = Bundle By Name(cluster=T6 {"dest_x"=0.0, "dest_y"=0.0, "dest_orientation"=0.0, "dest_vel"=0.0} ("element"), "dest_x"=w410, "dest_y"=w409, "dest_orientation"=w408) -> (w407:T6)
          n122 = Build Array(w407) -> (w406:T6[])
          n123 = Bundle By Name(cluster=w405, "Dest"=w406, "v_tangent"=w412, "v_normal"=w414, "v_ang"=w413, "kick_x"=0.0) -> (w404:T2)
        }
      }
    }
  }
  "Robot out" <- w21
  n124 = feedback-in #1(w26) -> ()
  n125 = feedback-in #2(w25) -> ()
